vi "Build Shared Library Search Path.vi"(8 "Error In":errorcluster, 11 "libssh2lv Shared Library":path=path "") -> (0 "Error Out":errorcluster, 3 "Search Path":path[](array[path]))   [LabVIEW 2018, in "Toolkit.lvlib" / "SSH.lvclass"]
doc: "Creates an array of paths, known as the \"Search Path\", to use to find a libssh2lv shared library."
uses:
  SSH.lvclass
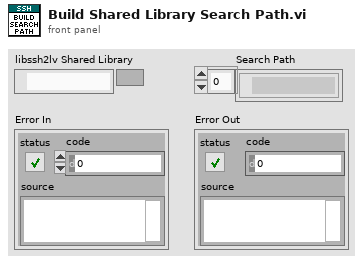
[diagram p1: front panel]
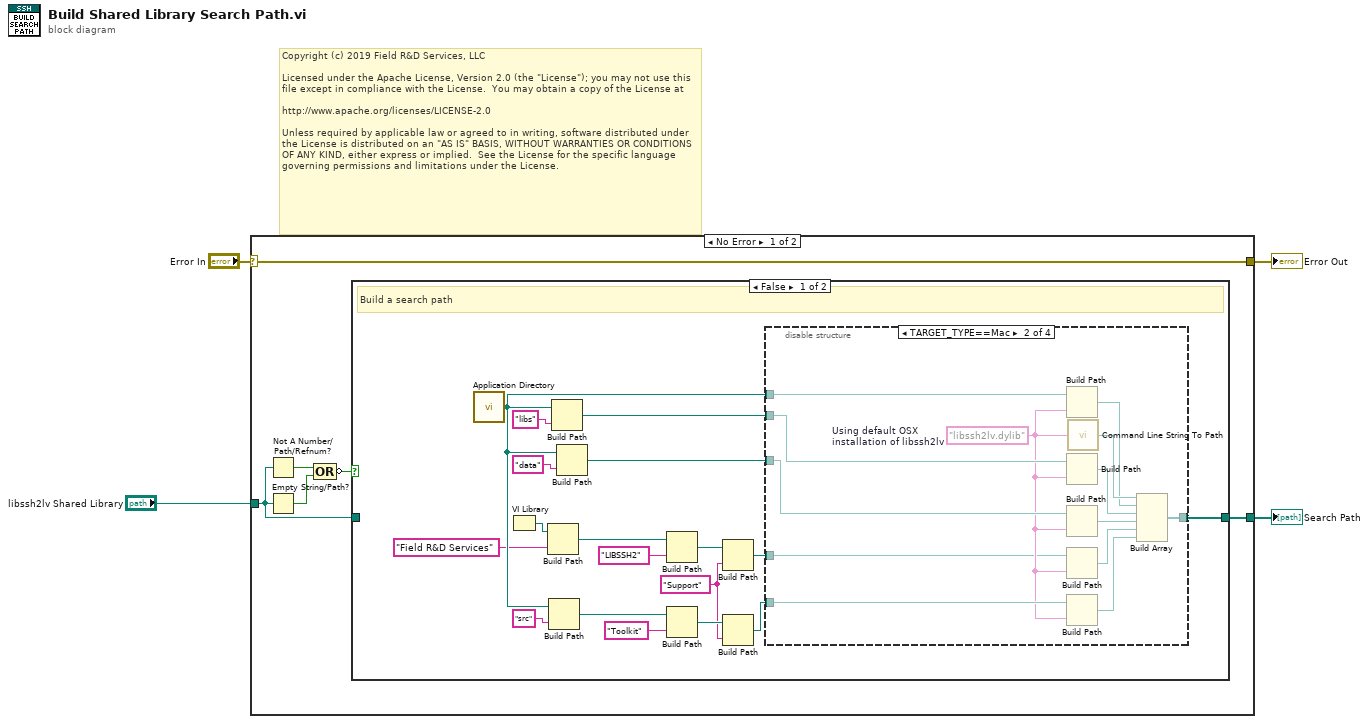
[diagram p0: block diagram]
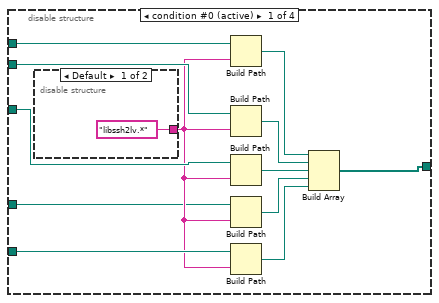
[diagram p2: hidden frame]
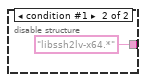
[diagram p3: hidden frame]
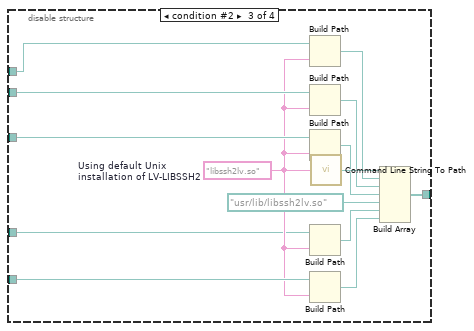
[diagram p4: hidden frame]
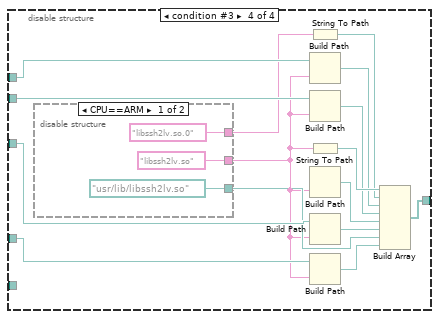
[diagram p5: hidden frame]
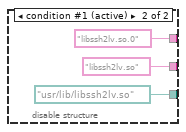
[diagram p6: hidden frame]
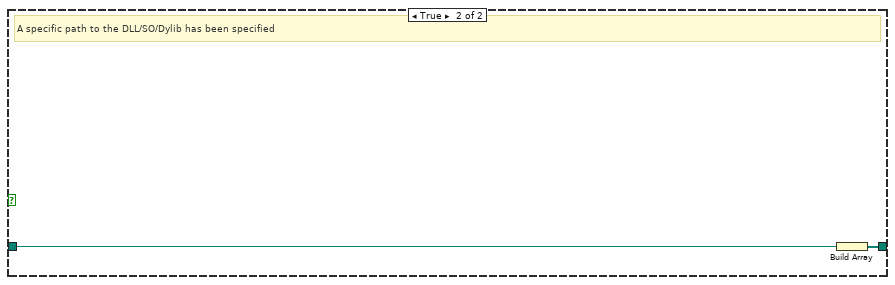
[diagram p7: hidden frame]
diagram:
  # "Copyright (c) 2019 Field R&D Services, LLC\n\nLicensed under the Apache License, Version 2.0 (the \"License\"); you may not use this file except in compliance with the License.  You may obtain a copy of the License at\n\nhttp://www.apache.org/licenses/LICENSE-2.0\n\nUnless required by applicable law or agreed to in writing, software distributed under the License is distributed on an \"AS IS\" BASIS, WITHOUT WARRANTIES OR CONDITIONS OF ANY KIND, either express or implied.  See the License for the specific language governing permissions and limitations under the License."
  n1 = case shown="No Error" "Error In" {
    selector: "Error In" -> [w9 w93]
    tunnel: [w10 _] -> w4
    tunnel: "libssh2lv Shared Library" -> [w6 _]
    tunnel: [w9 w93] -> w1
    frame No Error {
      n2 = Not A Number/Path/Refnum?(number/path/refnum=w6) -> (NaN/Path/Refnum?=w7:bool)
      n3 = Empty String/Path?(string/path=w6) -> (empty?=w8:bool)
      n4 = Compound Arithmetic op=OR(w7, w8) -> (invert w5:bool)
      n5 = case shown="False" w5 {
        tunnel: w6 -> [_ w92]
        tunnel: [w24 w91] -> w10
        frame False {
          w13 = "Support" ("name or relative path")
          # "Build a search path"
          n6 = call <vilib>:"Application Directory.vi"() -> ("Application Directory"=w22:path)
          n7 = VI Library() -> (path=w18:path)
          n8 = Build Path(base path=w18, name or relative path="Field R&D Services") -> (appended path=w16:path)
          n9 = Build Path ("EXE include\nlocation")(base path=w22, name or relative path="src") -> (appended path=w27:path)
          n10 = Build Path ("EXE include\nlocation")(base path=w22, name or relative path="libs") -> (appended path=w19:path)
          n11 = Build Path ("EXE include\nlocation")(base path=w22, name or relative path="data") -> (appended path=w20:path)
          n12 = Build Path(base path=w16, name or relative path="LIBSSH2") -> (appended path=w15:path)
          n13 = Build Path ("EXE include\nlocation")(base path=w27, name or relative path="Toolkit") -> (appended path=w28:path)
          n14 = Build Path(base path=w15, name or relative path=w13) -> (appended path=w14:path)
          n15 = Build Path ("EXE include\nlocation")(base path=w28, name or relative path=w13) -> (appended path=w25:path)
          n16 = disable-structure shown="TARGET_TYPE==Mac" {
            disable-tunnel: [w39 w54 w68 w84] -> w24
            disable-tunnel: w25 -> [w40 w53 w67 _]
            disable-tunnel: w22 -> [w38 w52 w62 w77]
            disable-tunnel: w19 -> [w37 w51 w61 w76]
            disable-tunnel: w20 -> [w36 w50 w60 w75]
            disable-tunnel: w14 -> [w34 w45 w58 w72]
            frame condition #0 (active) {
              n17 = disable-structure shown="Default" {
                disable-tunnel: ["libssh2lv.*" ("name or relative path") "libssh2lv-x64.*" ("name or relative path")] -> w35
                frame condition #0 (active) {
                }
                frame condition #1 {
                }
              }
              n18 = Build Path ("EXE include\nlocation")(base path=w38, name or relative path=w35) -> (appended path=w29:path)
              n19 = Build Path ("EXE include\nlocation")(base path=w37, name or relative path=w35) -> (appended path=w30:path)
              n20 = Build Path ("EXE include\nlocation")(base path=w36, name or relative path=w35) -> (appended path=w31:path)
              n21 = Build Path ("EXE include\nlocation")(base path=w34, name or relative path=w35) -> (appended path=w33:path)
              n22 = Build Path ("EXE include\nlocation")(base path=w40, name or relative path=w35) -> (appended path=w32:path)
              n23 = Build Array(w29, w30, w31, w33, w32) -> (w39:path[])
            }
            frame condition #1 {
              w46 = "libssh2lv.dylib"  # Using default OSX installation of libssh2lv
              n24 = Build Path ("EXE include\nlocation")(base path=w52, name or relative path=w46) -> (appended path=w49:path)
              n25 = Build Path ("EXE include\nlocation")(base path=w51, name or relative path=w46) -> (appended path=w48:path)
              n26 = Build Path ("EXE include\nlocation")(base path=w50, name or relative path=w46) -> (appended path=w47:path)
              n27 = Build Path ("EXE include\nlocation")(base path=w45, name or relative path=w46) -> (appended path=w44:path)
              n28 = Build Path ("EXE include\nlocation")(base path=w53, name or relative path=w46) -> (appended path=w43:path)
              n29 = call <vilib>:"Command Line String To Path.vi"("string"=w46) -> ("path"=w55:path)
              n30 = Build Array(w55, w49, w48, w47, w44, w43) -> (w54:path[])
            }
            frame condition #2 {
              w59 = "libssh2lv.so"  # Using default Unix installation of LV-LIBSSH2
              n31 = Build Path ("EXE include\nlocation")(base path=w62, name or relative path=w59) -> (appended path=w65:path)
              n32 = Build Path ("EXE include\nlocation")(base path=w61, name or relative path=w59) -> (appended path=w64:path)
              n33 = Build Path ("EXE include\nlocation")(base path=w60, name or relative path=w59) -> (appended path=w63:path)
              n34 = Build Path ("EXE include\nlocation")(base path=w58, name or relative path=w59) -> (appended path=w57:path)
              n35 = Build Path ("EXE include\nlocation")(base path=w67, name or relative path=w59) -> (appended path=w56:path)
              n36 = call <vilib>:"Command Line String To Path.vi"("string"=w59) -> ("path"=w69:path)
              n37 = Build Array(w69, w65, w64, w63, path "/usr/lib/libssh2lv.so" ("path"), w57, w56) -> (w68:path[])
            }
            frame condition #3 {
              n38 = disable-structure "Conditional Disable Structure" shown="CPU==ARM" {
                disable-tunnel: ["libssh2lv.so.0" "libssh2lv.so.0"] -> w74
                disable-tunnel: ["libssh2lv.so" "libssh2lv.so"] -> w71
                disable-tunnel: [path "/usr/lib/libssh2lv.so" ("path") path "/usr/lib/libssh2lv.so" ("path")] -> w73
                frame condition #0 {
                }
                frame condition #1 (active) {
                }
              }
              n39 = String To Path(string=w74) -> (path=w82:path)
              n40 = Build Path ("EXE include\nlocation")(base path=w77, name or relative path=w71) -> (appended path=w78:path)
              n41 = Build Path ("EXE include\nlocation")(base path=w76, name or relative path=w71) -> (appended path=w81:path)
              n42 = String To Path(string=w71) -> (path=w83:path)
              n43 = Build Path ("EXE include\nlocation")(name or relative path=w71) -> (appended path=w80:path)  [unwired: 1 in]
              n44 = Build Path ("EXE include\nlocation")(base path=w75, name or relative path=w71) -> (appended path=w79:path)
              n45 = Build Path ("EXE include\nlocation")(base path=w72, name or relative path=w71) -> (appended path=w70:path)
              n46 = Build Array(w83, w82, w78, w81, w80, w79, w73, w70) -> (w84:path[])
            }
          }
        }
        frame True {
          # "A specific path to the DLL/SO/Dylib has been specified"
          n47 = Build Array(w92) -> (w91:path[])
        }
      }
    }
    frame Error {
    }
  }
  "Search Path" <- w4
  "Error Out" <- w1
